vi "setTitle.vi"(7 "Offset":cluster{"horizontal":dbl, "vertical":dbl}, 8 "Set?":bool=TRUE, 9 "Title":string, 11 "String in":string) -> (2 "command":string, 3 "String out":string)   [LabVIEW 2012]
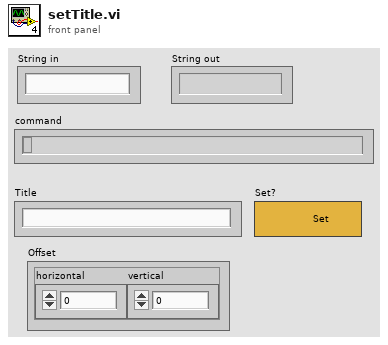
[diagram p1: front panel]
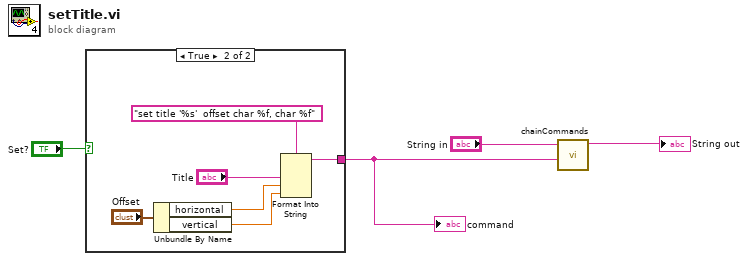
[diagram p0: block diagram]
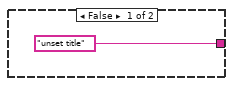
[diagram p2: hidden frame]
diagram:
  n1 = case shown="True" "Set?" {
    tunnel: ["unset title" w10] -> w3
    frame False {
    }
    frame True {
      n2 = Unbundle By Name("Offset") -> ("horizontal"=w7:dbl, "vertical"=w6:dbl)
      n3 = Format Into String(format string="set title '%s'  offset char %f, char %f", "Title", w7, w6) -> (resulting string=w10:string)  [unwired: 2 in, 1 out]
    }
  }
  "command" <- w3
  n4 = call "chainCommands.vi"("Command"=w3, "StringIn"="String in") -> ("StringOut"=→"String out":string)  [unwired: 9 in]
